vi "tempconfigAI_seal.vi"(1 "Temp Config in":T2, 2 "command":string) -> (0 "Temp Config out":T1)   [LabVIEW 2015]
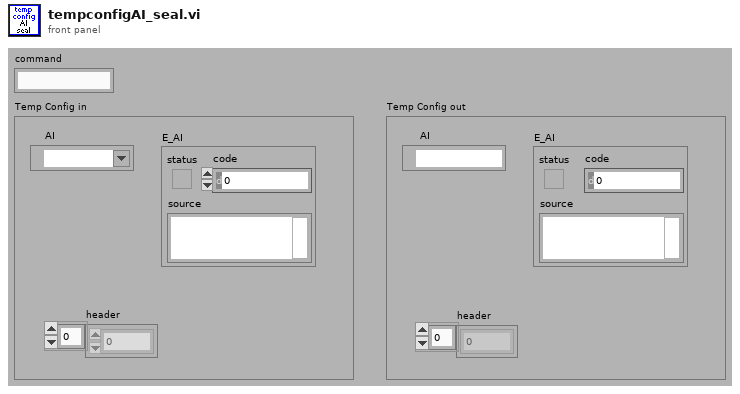
[diagram p1: front panel]
types:
  T1 = cluster{" AI":refnum<k21>, "E_AI":errorcluster, "header":dbl[]}
  T2 = cluster{"AI":refnum<k21>, "E_AI":errorcluster, "header":dbl[]}
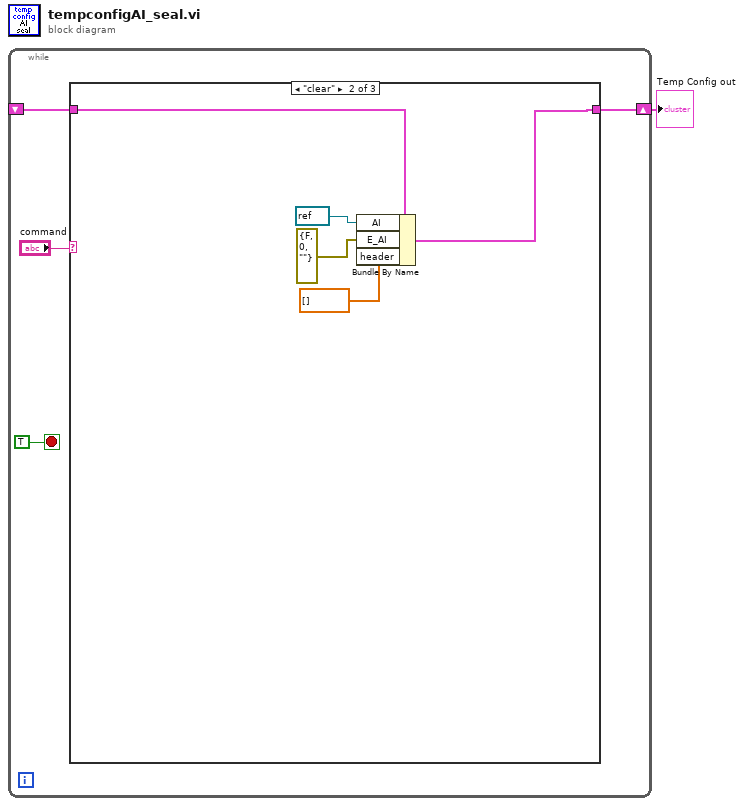
[diagram p0: block diagram]
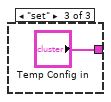
[diagram p3: hidden frame]
diagram:
  n1 = while {
    shift-right: [w3] -> w1
    shift-left: _ -> [w2]
    stop <- TRUE stop-if-true
    n2 = case shown="\"clear\"" "command" {
      tunnel: [w6 w8 "Temp Config in"] -> w3
      tunnel: w2 -> [w6 w11 _]
      frame "get", Default {
      }
      frame "clear" {
        n3 = Bundle By Name(cluster=w11, "AI"=refnum<k21> refnum ("XY"), "E_AI"=errorcluster {"status"=FALSE, "code"=0, "source"=""}, "header"=dbl[] []) -> (w8:T2)
      }
      frame "set" {
      }
    }
  }
  "Temp Config out" <- w1
